vi "Configure Spectrum Emission Mask (Offset Frequency).vi"(0 "VISA resource name":refnum<visa-resource-name>, 5 "SEM Start Frequency":dbl[](array[numeric]) min=10000.0 max=500000000.0, 7 "SEM Stop Frequency":dbl[](array[numeric]) min=10000.0 max=500000000.0, 11 "error in (no error)":errorcluster) -> (4 "VISA resource name out":refnum<visa-resource-name>, 15 "error out":errorcluster)   [LabVIEW 2020, in "Anritsu Signal Analyzer Series.lvlib"]
doc: "Configures the setup for offset frequency of SEM measurement settings of the spectrum analyzer."
uses:
  Anritsu Signal Analyzer Series.lvlib
panel:
  # "Hz"
  # "Hz"
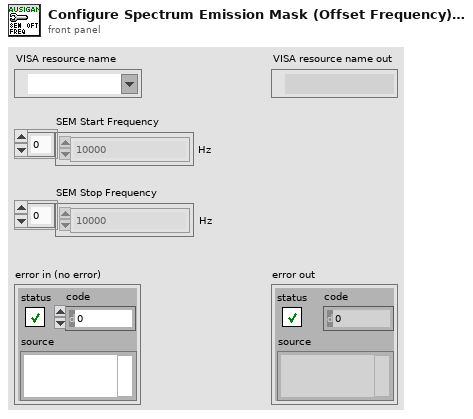
[diagram p1: front panel]
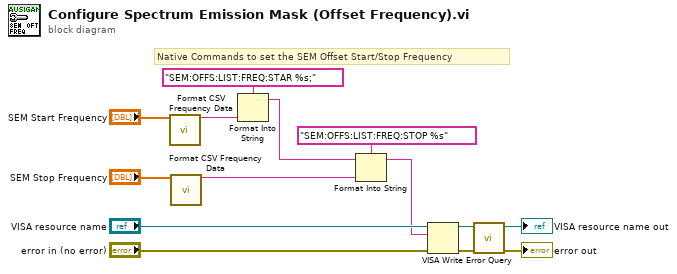
[diagram p0: block diagram]
diagram:
  # "Native Commands to set the SEM Offset Start/Stop Frequency"
  n1 = call "Format CSV Frequency Data.vi"("Data_In"="SEM Start Frequency") -> ("Data_out"=w4:string)  [unwired: 14 in]
  n2 = call "Format CSV Frequency Data.vi"("Data_In"="SEM Stop Frequency") -> ("Data_out"=w3:string)  [unwired: 14 in]
  n3 = Format Into String(format string="SEM:OFFS:LIST:FREQ:STAR %s;" ("_CommandSet"), w4) -> (resulting string=w7:string)  [unwired: 2 in, 1 out]
  n4 = Format Into String(format string="SEM:OFFS:LIST:FREQ:STOP %s" ("_CommandSet"), initial string=w7, w3) -> (resulting string=w5:string)  [unwired: 1 in, 1 out]
  n5 = VISA Write(VISA resource name="VISA resource name", write buffer=w5, error in (no error)="error in (no error)") -> (VISA resource name out=w1:refnum<visa-resource-name>, error out=w2:errorcluster)  [unwired: 1 out]
  n6 = call "Error Query.vi"("error in (no error)"=w2, "VISA resource name"=w1) -> ("error out"=→"error out":errorcluster, "VISA resource name out"=→"VISA resource name out":refnum<visa-resource-name>)  [unwired: 6 in, 2 out]
